vi "SCP Close.vi"(8 "Error In":errorcluster, 11 "SCP Session":refnum<k24>) -> (0 "Error Out":errorcluster)   [LabVIEW 2014, in "LMH-LINX.lvlib"]
uses:
  <vilib>/MakerHub/LINX/LMH-LINX.lvlib
  C:/Program Files (x86)/National Instruments/LabVIEW 2014/vi.lib/MakerHub/LINX/Resources/Renci.SshNet.dll
  Resources/Renci.SshNet.dll
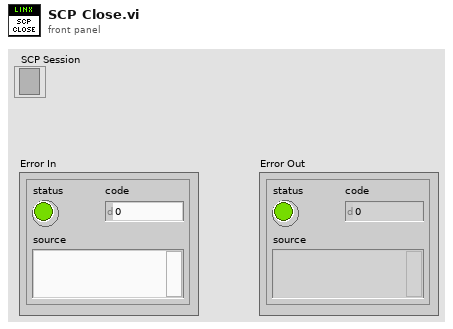
[diagram p1: front panel]
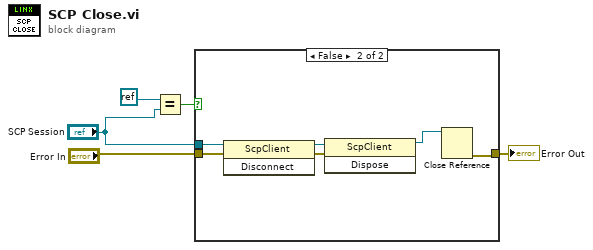
[diagram p0: block diagram]
diagram:
  n1 = Equal?(x=refnum<k0> refnum, y="SCP Session") -> (x = y?=w1:bool)
  n2 = case shown="False" w1 {
    tunnel: [w6 w7] -> w5
    tunnel: "Error In" -> [w6 w10]
    tunnel: "SCP Session" -> [_ w9]
    frame True {
    }
    frame False {
      n3 = invoke class="ScpClient" method="Disconnect"(reference=w9, error in=w10) -> (reference out=w12:refnum<k24>, error out=w11:errorcluster)  [unwired: 1 in, 1 out]
      n4 = invoke class="ScpClient" method="Dispose"(reference=w12, error in=w11) -> (reference out=w8:refnum<k24>)  [unwired: 1 in, 2 out]
      n5 = Close Reference(reference=w8) -> (error out=w7:errorcluster)  [unwired: 1 in]
    }
  }
  "Error Out" <- w5
